vi "estimate current pos and vel kalman.vi"(9 "feedback lowpass f":dbl=30.0 format="%0.4f", 11 "kalman updates":T1[](array[typedef])) -> (4 "current velocity":dbl[](array[numeric]), 5 "current position":dbl[](array[numeric]))   [LabVIEW 2010]
uses:
  kalman_result_scaled.ctl
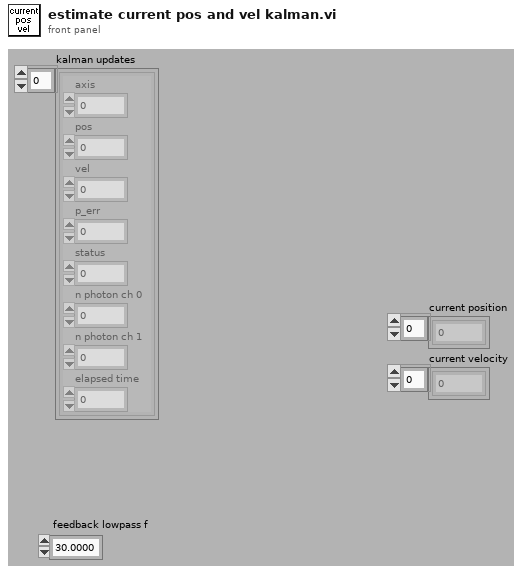
[diagram p1: front panel]
types:
  T1 = typedef "kalman_result_scaled.ctl" = cluster{"axis":u8, "pos":dbl, "vel":dbl, "p_err":dbl, "status":u32, "n photon ch 0":u32, "n photon ch 1":u32, "elapsed time":dbl}
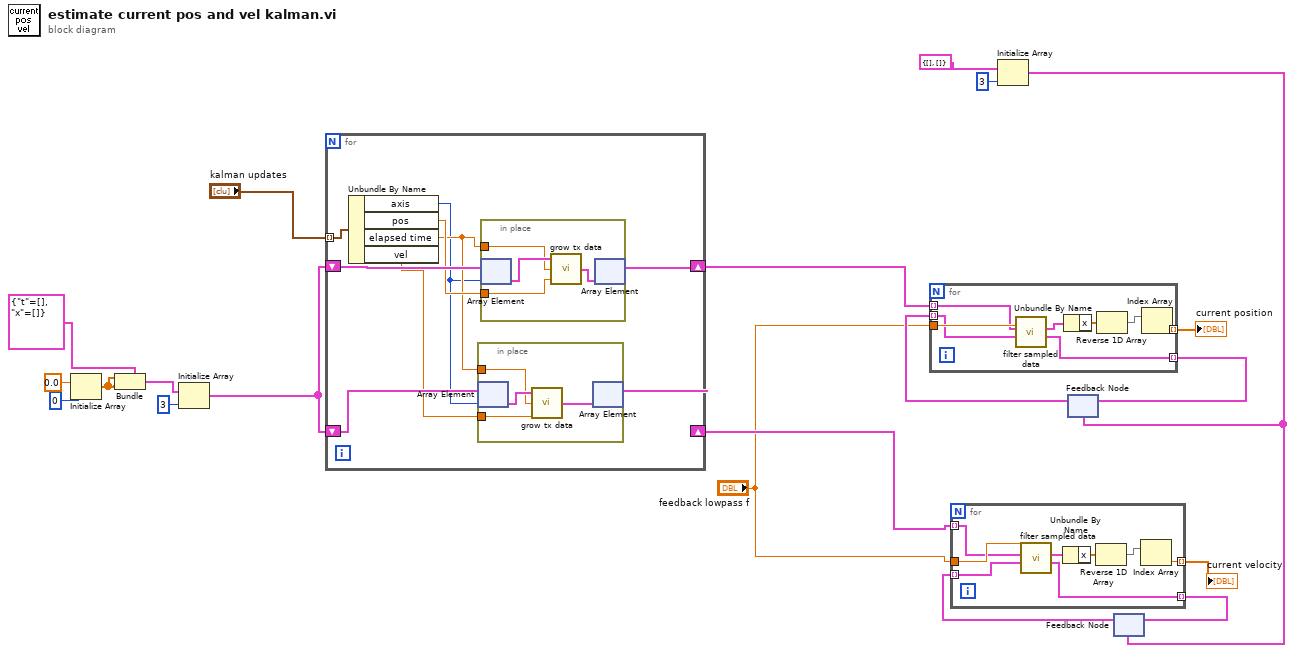
[diagram p0: block diagram]
diagram:
  n1 = Initialize Array(0.0 ("element"), 0 ("dimension size")) -> (w13:dbl[])
  n2 = Bundle(cluster=cluster{"t":dbl[], "x":dbl[]} {"t"=[], "x"=[]} ("xt val"), "t"=w13, "x"=w13) -> (w6:cluster{"t":dbl[], "x":dbl[]})
  n3 = Initialize Array(w6, 3 ("dimension size")) -> (w19:cluster{"t":dbl[], "x":dbl[]}[])
  n4 = for {
    tunnel: "kalman updates" -> [w21] mode=indexing
    shift-right: [w27] -> w5
    shift-left: w19 -> [w29]
    shift-right: [w22] -> w18
    shift-left: w19 -> [w26]
    n5 = Unbundle By Name(w21) -> ("axis"=w23:u8, "pos"=w28:dbl, "elapsed time"=w25:dbl, "vel"=w24:dbl)
    n6 = in-place {
      in-place-border: w25 -> [w32]
      in-place-border: w24 -> [w31]
      n7 = in-place-array #1(w26, w23) -> (w33:cluster{"t":dbl[], "x":dbl[]})
      n8 = call "grow tx data.vi"("value"=w31, "time"=w32, "tx data in"=w33) -> ("tx data out"=w30:cluster{"t":dbl[], "x":dbl[]})
      n9 = in-place-array #1(w30) -> (w22:cluster{"t":dbl[], "x":dbl[]}[])  [unwired: 1 out]
    }
    n10 = in-place {
      in-place-border: w25 -> [w36]
      in-place-border: w28 -> [w35]
      n11 = in-place-array #2(w29, w23) -> (w37:cluster{"t":dbl[], "x":dbl[]})
      n12 = call "grow tx data.vi"("value"=w35, "time"=w36, "tx data in"=w37) -> ("tx data out"=w34:cluster{"t":dbl[], "x":dbl[]})
      n13 = in-place-array #2(w34) -> (w27:cluster{"t":dbl[], "x":dbl[]}[])  [unwired: 1 out]
    }
  }
  n14 = Initialize Array(cluster{"t":dbl[], "x":dbl[]} {"t"=[], "x"=[]} ("xt val"), 3 ("dimension size")) -> (w7:cluster{"t":dbl[], "x":dbl[]}[])
  n15 = feedback #3(w7) -> (w10:cluster{"t":dbl[], "x":dbl[]}[])
  n16 = for {
    tunnel: w5 -> [w44] mode=indexing
    tunnel: [w38] -> w11 mode=indexing
    tunnel: w10 -> [w43] mode=indexing
    tunnel: "feedback lowpass f" -> [w45]
    tunnel: [w39] -> w4 mode=indexing
    n17 = call "filter sampled data.vi"("low cutoff freq: fl"=w45, "last data set"=w43, "t x data"=w44) -> ("current data set"=w38:cluster{"t":dbl[], "x":dbl[]}, "t x data filetered"=w42:cluster{"t":dbl[], "x":dbl[]})  [unwired: 7 in]
    n18 = Unbundle By Name(w42) -> ("x"=w40:dbl[])
    n19 = Reverse 1D Array(array=w40) -> (reversed array=w41:dbl[])
    n20 = Index Array(array=w41) -> (element=w39:dbl)  [unwired: 1 in]
  }
  "current position" <- w4
  n21 = feedback-in #3(w11) -> ()
  n22 = feedback #4(w7) -> (w8:cluster{"t":dbl[], "x":dbl[]}[])
  n23 = for {
    tunnel: w18 -> [w52] mode=indexing
    tunnel: [w46] -> w9 mode=indexing
    tunnel: w8 -> [w51] mode=indexing
    tunnel: "feedback lowpass f" -> [w53]
    tunnel: [w47] -> w2 mode=indexing
    n24 = call "filter sampled data.vi"("low cutoff freq: fl"=w53, "last data set"=w51, "t x data"=w52) -> ("current data set"=w46:cluster{"t":dbl[], "x":dbl[]}, "t x data filetered"=w48:cluster{"t":dbl[], "x":dbl[]})  [unwired: 7 in]
    n25 = Unbundle By Name(w48) -> ("x"=w49:dbl[])
    n26 = Reverse 1D Array(array=w49) -> (reversed array=w50:dbl[])
    n27 = Index Array(array=w50) -> (element=w47:dbl)  [unwired: 1 in]
  }
  "current velocity" <- w2
  n28 = feedback-in #4(w9) -> ()
